vi "count_until_N.vi"(10 "N":u8=74) -> (1 "counter":u8, 3 "turn around !":bool)   [LabVIEW 2018, in "tools.lvlib"]
uses:
  tools.lvlib
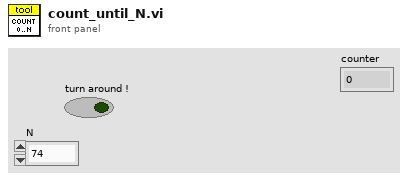
[diagram p1: front panel]
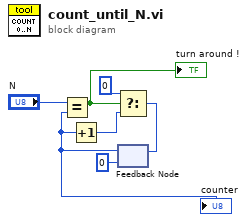
[diagram p0: block diagram]
diagram:
  n1 = feedback #1(i16 0) -> (w6:i16)
  "counter" <- w6
  n2 = Equal?(x="N", y=w6) -> (x = y?=w7:bool)
  "turn around !" <- w7
  n3 = Increment(x=w6) -> (x+1=w4:i16)
  n4 = Select(t=i16 0, s=w7, f=w4) -> (s? t:f=w3:i16)
  n5 = feedback-in #1(w3) -> ()
